vi "Add Task.vi"(8 "error in (no error)":errorcluster, 10 "Digital Configuration Parameters":T1, 11 "Digital Input in":refnum<class "Digital Input.lvclass">) -> (0 "error out":errorcluster, 3 "Digital Input out":refnum<class "Digital Input.lvclass">)   [LabVIEW 2021, in "Digital Input.lvclass"]
uses:
  Digital Input.lvclass
  Digital Input.lvclass/Digital Input.ctl
  <resource>/objmgr/daqmx.rc
  <vilib>/DAQmx/create/channels.llb/DAQmx Create Channel (DI-Digital Input).vi
  Utilities/Digital Configuration Parameters.ctl
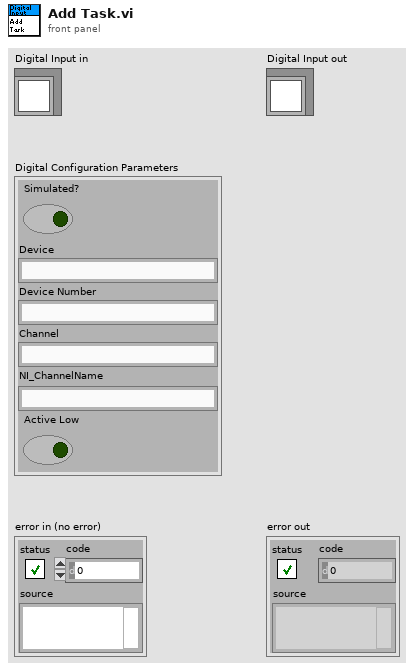
[diagram p1: front panel]
types:
  T1 = typedef "Digital Configuration Parameters.ctl" = cluster{"Simulated?":bool, "Device":string, "Device Number":string, "Channel":string, "NI_ChannelName":string, "Active Low":bool}
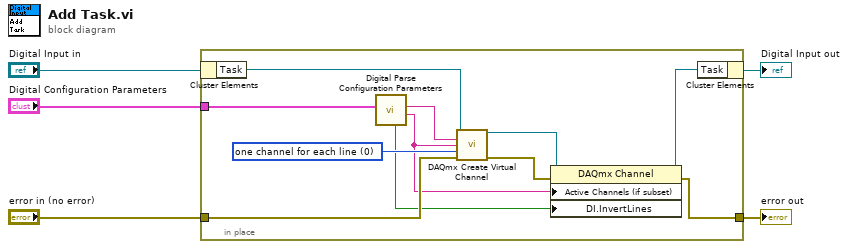
[diagram p0: block diagram]
diagram:
  n1 = in-place {
    in-place-border: "Digital Configuration Parameters" -> [w11]
    in-place-border: "error in (no error)" -> [w9]
    in-place-border: [w8] -> w1
    w15 = 0 items=["one channel for each line", "one channel for all lines"] ("line grouping")
    n2 = in-place-cluster #1("Digital Input in") -> ("Task"=w16:refnum<k21>)
    n3 = call "Digital Parse Configuration Parameters.vi"("Digital Configuration Parameters"=w11) -> ("name to assign"=w7:string, "lines"=w10:string, "Active Low"=w6:bool)  [unwired: 8 in]
    n4 = call-poly <vilib>:"DAQmx Create Virtual Channel.vi"("task in"=w16, "lines"=w10, "name to assign"=w7, "line grouping"=w15, "error in"=w9) -> ("task out"=w14:refnum<k21>, "error out"=w12:errorcluster)  [unwired: 9 in]
    n5 = property class="DAQmx Channel"(reference=w14, error in=w12, "Active Channels (if subset)"=w7, "DI.InvertLines"=w6) -> (reference out=w13:refnum<k21>, error out=w8:errorcluster)
    n6 = in-place-cluster #1("Task"=w13) -> (→"Digital Input out":refnum<class "Digital Input.lvclass">)
  }
  "error out" <- w1
